vi "Elevator State Select.vi"() -> ()   [LabVIEW 2018]
uses:
  RefNumsDriverStation.vi
  Users/marka/Desktop/Secret City Wildbots Summer Project/2019_Robot_Project/2019 Summer Rebuild/Robot States.vi
panel:
  out "Elevator_State":string
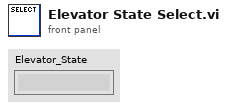
[diagram p1: front panel]
types:
  T1 = cluster{"Elevator_Stow":bool, "Cargo_Rocket_1":bool, "Hatch_Rocket_1":bool, "Cargo_Ground":bool, "Hatch_Feeder":bool, "Cargo_Ship":bool, "Hatch_Ship":bool}
  T2 = cluster{"Trigger":bool, "Trigger":bool, "Trigger":bool, "Trigger":bool, "Trigger":bool, "Trigger":bool, "Trigger":bool}
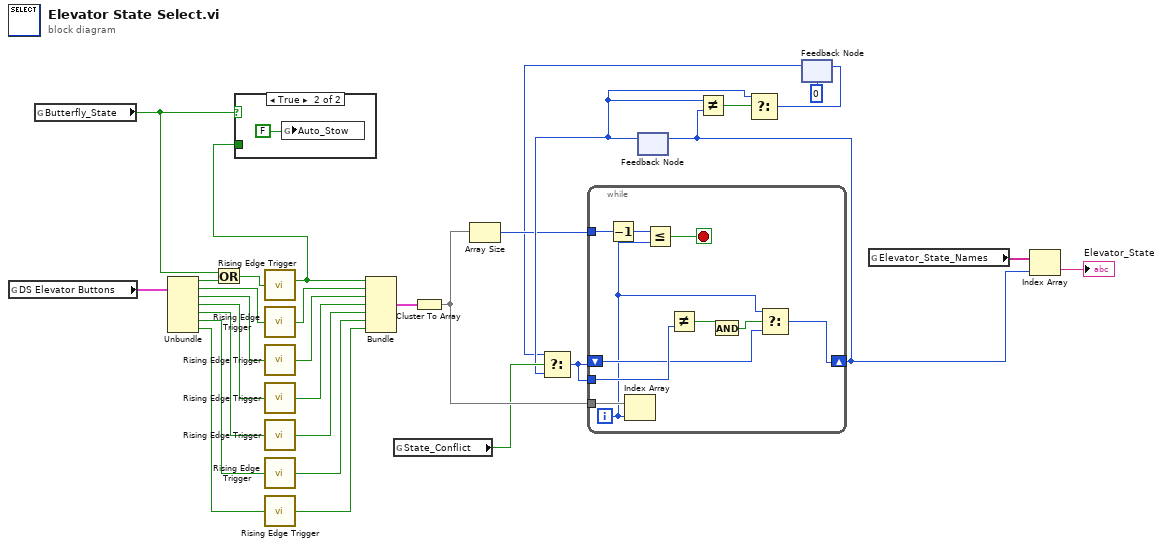
[diagram p0: block diagram]
diagram:
  n1 = global read "RefNumsDriverStation.vi" "DS Elevator Buttons"() -> (w30:T1)
  n2 = global read "Robot States.vi" "Butterfly_State"() -> (w14:bool)
  n3 = Unbundle(w30) -> ("Elevator_Stow"=w16:bool, "Cargo_Rocket_1"=w29:bool, "Hatch_Rocket_1"=w28:bool, "Cargo_Ground"=w27:bool, "Hatch_Feeder"=w26:bool, "Cargo_Ship"=w25:bool, "Hatch_Ship"=w24:bool)
  n4 = Or(x=w14, y=w16) -> (x .or. y?=w15:bool)
  n5 = call "Rising Edge Trigger.vi"("Raw Signal"=w15) -> ("Trigger"=w13:bool)
  n6 = case shown="True" w14 {
    tunnel: w13 -> [_ _]
    frame False {
    }
    frame True {
      n7 = global write "Robot States.vi" "Auto_Stow"(FALSE ("Auto_Stow")) -> ()
    }
  }
  n8 = call "Rising Edge Trigger.vi"("Raw Signal"=w29) -> ("Trigger"=w23:bool)
  n9 = call "Rising Edge Trigger.vi"("Raw Signal"=w28) -> ("Trigger"=w22:bool)
  n10 = call "Rising Edge Trigger.vi"("Raw Signal"=w27) -> ("Trigger"=w21:bool)
  n11 = call "Rising Edge Trigger.vi"("Raw Signal"=w26) -> ("Trigger"=w20:bool)
  n12 = call "Rising Edge Trigger.vi"("Raw Signal"=w25) -> ("Trigger"=w19:bool)
  n13 = call "Rising Edge Trigger.vi"("Raw Signal"=w24) -> ("Trigger"=w18:bool)
  n14 = Bundle("Trigger"=w13, "Trigger"=w23, "Trigger"=w22, "Trigger"=w21, "Trigger"=w20, "Trigger"=w19, "Trigger"=w18) -> (w17:T2)  [unwired: 1 in]
  n15 = global read "Robot States.vi" "State_Conflict"() -> (w11:bool)
  n16 = Cluster To Array(cluster=w17) -> (array=w12:bool[])
  n17 = Array Size(array=w12) -> (size(s)=w7:i32)
  n18 = feedback #1() -> (w9:i32)  [unwired: 1 in]
  n19 = feedback #2(0) -> (w3:i32)
  n20 = Select(t=w3, s=w11, f=w9) -> (s? t:f=w8:i32)
  n21 = while {
    tunnel: w12 -> [w41]
    shift-right: [w32] -> w6
    shift-left: w8 -> [w34]
    tunnel: w8 -> [w38]
    tunnel: w7 -> [w37]
    i -> [w33]
    stop <- w35 stop-if-true
    n22 = Decrement(x=w37) -> (x-1=w36:i32)
    n23 = Index Array(array=w41, index=w33) -> ()  [unwired: 1 out]
    n24 = Less Or Equal?(x=w36, y=w33) -> (x <= y?=w35:bool)
    n25 = Not Equal?(y=w38) -> (x != y?=w40:bool)  [unwired: 1 in]
    n26 = And(x=w40) -> (x .and. y?=w39:bool)  [unwired: 1 in]
    n27 = Select(t=w33, s=w39, f=w34) -> (s? t:f=w32:i32)
  }
  n28 = feedback-in #1(w6) -> ()
  n29 = Not Equal?(x=w9, y=w6) -> (x != y?=w10:bool)
  n30 = Select(t=w9, s=w10) -> (s? t:f=w5:i32)  [unwired: 1 in]
  n31 = feedback-in #2(w5) -> ()
  n32 = global read "Robot States.vi" "Elevator_State_Names"() -> (w2:string[])
  n33 = Index Array(array=w2, index=w6) -> (element=→"Elevator_State":string)
